vi "Image Sharpness Indicator.vi"() -> ()   [LabVIEW 2020]
uses:
  <vilib>/Platform/TimedLoop/XDataNode/timing_clust.ctl
  <vilib>/Platform/TimedLoop/XDataNode/nitl_modes.ctl
  <vilib>/Platform/TimedLoop/XDataNode/wakeup.ctl
  <vilib>/platform/TimedLoop/XDataNode/XDataNode.xnode
  <vilib>/Platform/TimedLoop/XDataNode/XDNodeRunTimeDep.lvlib
  <vilib>/MakerHub/Toolbox/LMH-Toolbox.lvlib
panel:
  out "Microscope Image":picture
  out "path to PNG file":path
  out "Waveform Graph":dbl[][](graph)
  out "Intensity Graph 2":dbl[][](graph)
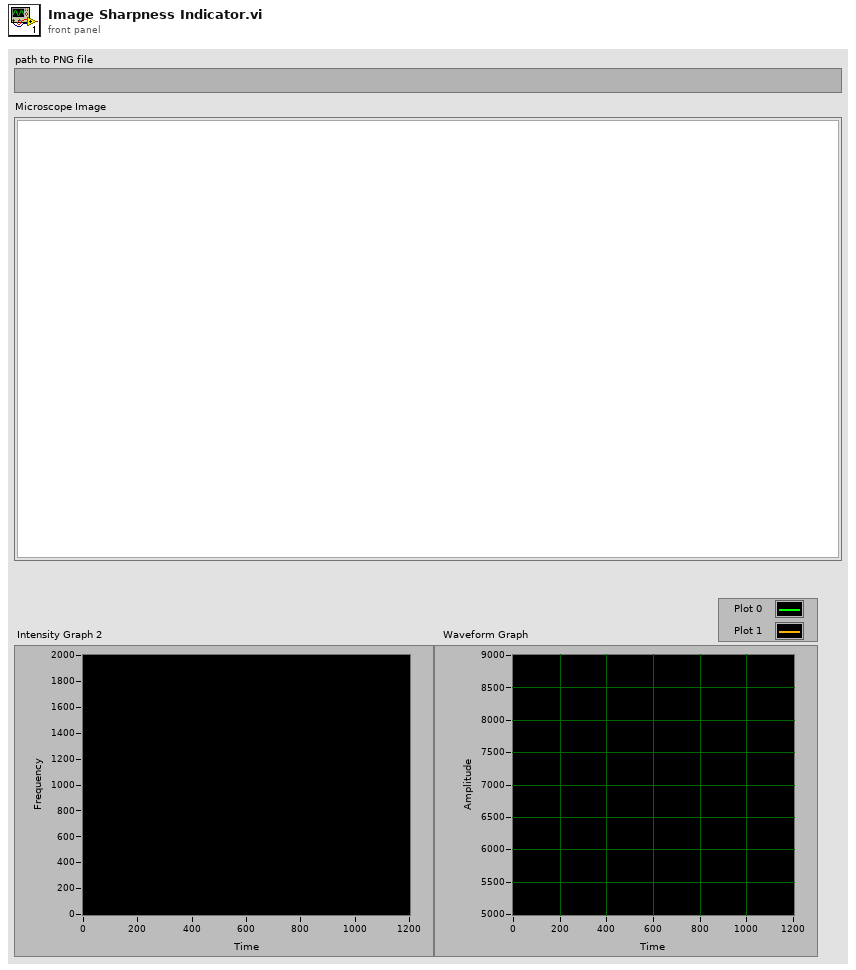
[diagram p1: front panel]
types:
  T1 = typedef "XDNodeRunTimeDep.lvlib/timing_clust.ctl" = cluster{"Expected End [f-1]":u64, "Actual End [f-1]":u64, "Finished Late? [f-1]":bool, "Expected End [i-1]":u64, "Actual End [i-1]":u64, "Finished Late? [i-1]":bool, "Expected Start [i]":u64, "Actual Start [i]":u64, "Expected Start [f]":u64, "Actual Start [f]":u64, "Source Name":string, "Structure Name":string, "Period":i64, "Deadline":i64, "Offset":i64, "Start":i64, "Priority":i32, "Timeout":i32, "Mode":T2, "Wakeup Reason":T3, "Error":errorcluster, "Source Type":string, "Secondary Source Type":string, "Global End Time":u64, "Global Start Time":u64, "Frame Duration":u64, "Iteration Duration":u64, "Assigned CPU":i32, "I/O Scan Engine Mode":u32}
  T2 = typedef "XDNodeRunTimeDep.lvlib/nitl_modes.ctl" = enum32{"No Change", "Process missed periods, maintain original phase", "Discard missed periods, maintain original phase", "Process missed periods, ignore original phase", "Discard missed periods, ignore original phase"}
  T3 = typedef "XDNodeRunTimeDep.lvlib/wakeup.ctl" = enum32{"Normal", "Aborted", "Asynchronous wakeup", "Timing source error", "Timed loop error", "Timeout"}
  T4 = typedef "imagedata.ctl" = cluster{"image type":i32, "image depth":i32, "image":u8[], "mask":u8[], "colors":u32[], "Rectangle":cluster{"left":i16, "top":i16, "right":i16, "bottom":i16}}
  T5 = typedef "LVBoundsTypeDef.ctl" = cluster{"Width":u32, "Height":u32}
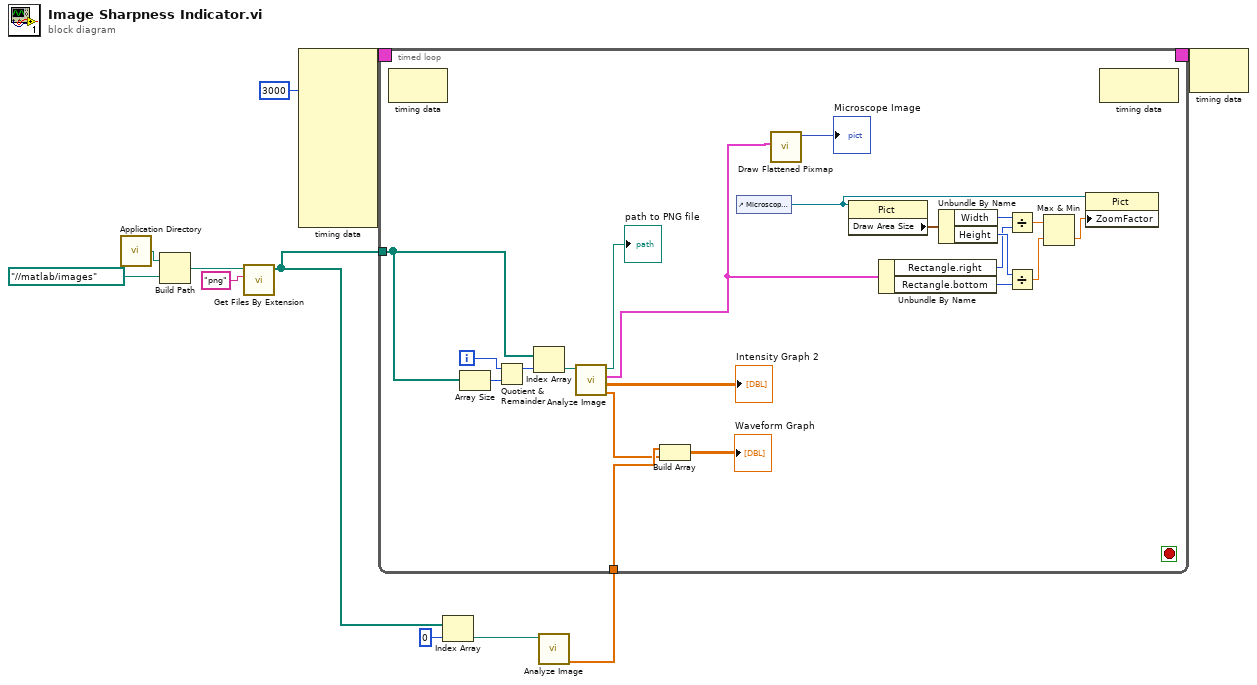
[diagram p0: block diagram]
diagram:
  n1 = call <vilib>:"Application Directory.vi"() -> ("Application Directory"=w11:path)
  n2 = Build Path(base path=w11, name or relative path=path "../../matlab/images") -> (appended path=w7:path)
  n3 = call <vilib>:"Get Files By Extension.vi"("Extention"="png", "Directory"=w7) -> ("Files With Extension"=w4:path[])  [unwired: 8 in, 1 out]
  n4 = node-c288(i64 3000 ("Period")) -> (w9:T1)  [unwired: 9 in]
  n5 = Index Array(array=w4, index=0) -> (element=w2:path)
  n6 = call "Analyze Image.vi"("path to PNG file"=w2) -> ("Log Sums"=w1:dbl[])  [unwired: 7 in, 3 out]
  n7 = timed-loop {
    timing: w9 -> [_]
    timing-out: [_] -> w8
    tunnel: w4 -> [w32]
    tunnel: w1 -> [w13]
    i -> [w30]
    stop <- _ stop-if-true
    n8 = node-c288() -> ()  [unwired: 1 in, 1 out]
    n9 = Array Size(array=w32) -> (size(s)=w31:i32)
    n10 = Quotient & Remainder(x=w30, y=w31) -> (x-y*floor(x/y)=w29:i32)  [unwired: 1 out]
    n11 = Index Array(array=w32, index=w29) -> (element=w28:path)
    n12 = call "Analyze Image.vi"("path to PNG file"=w28) -> ("Log Sums"=w12:dbl[], "2D FFT"=→"Intensity Graph 2":dbl[][], "image data"=w17:T4, "path to PNG file"=→"path to PNG file":path)  [unwired: 7 in]
    n13 = Build Array(w13, w12) -> (→"Waveform Graph":dbl[][])
    n14 = control-ref of="Microscope Image"() -> (w20:refnum<vi>)
    n15 = call <vilib>:"Draw Flattened Pixmap.vi"("image data"=w17) -> ("new picture"=→"Microscope Image":picture)  [unwired: 8 in]
    n16 = property class="Pict"(reference=w20) -> ("Draw Area Size"=w25:T5)  [unwired: 1 in, 2 out]
    n17 = Unbundle By Name(w17) -> ("Rectangle.right"=w16:i16, "Rectangle.bottom"=w15:i16)
    n18 = Unbundle By Name(w25) -> ("Width"=w24:u32, "Height"=w23:u32)
    n19 = Divide(x=w24, y=w16) -> (x/y=w22:dbl)
    n20 = Divide(x=w23, y=w15) -> (x/y=w21:dbl)
    n21 = Max & Min(x=w22, y=w21) -> (min(x,y)=w19:dbl)  [unwired: 1 out]
    n22 = property class="Pict"(reference=w20, "ZoomFactor"=w19) -> ()  [unwired: 1 in, 2 out]
    n23 = node-c288() -> ()  [unwired: 1 in, 1 out]
  }
  n24 = node-c288(w8) -> ()  [unwired: 1 out]
